vi "Create Startup CDF (Software Set).vi"(3 "Application Path":path, 4 "Add-ons":T1[](array[typedef]) {"component type" items=["standard", "hidden", "system", "unknown", "startup", "image", "essential"]}, 5 "Device Class":string, 6 "Software Set":T1 {"component type" items=["standard", "hidden", "system", "unknown", "startup", "image", "essential"]}, 7 "Operating System":string, 8 "error in (no error)":errorcluster, 9 "Files":path[](array[path]), 10 "Application Info":T1={"title"="", "description"="", "ID"="", "version"="", "component type"=4} {"component type" items=["standard", "hidden", "system", "unknown", "startup", "image", "essential"]}, 11 "CDF Location":path) -> (0 "error out":errorcluster)   [LabVIEW 2017, in "nisyscfg.lvlib"]
uses:
  <vilib>/nisyscfg/nisyscfg.lvlib
  <vilib>/nisyscfg/Software 1.2.ctl
  <vilib>/nisyscfg/Component Type.ctl
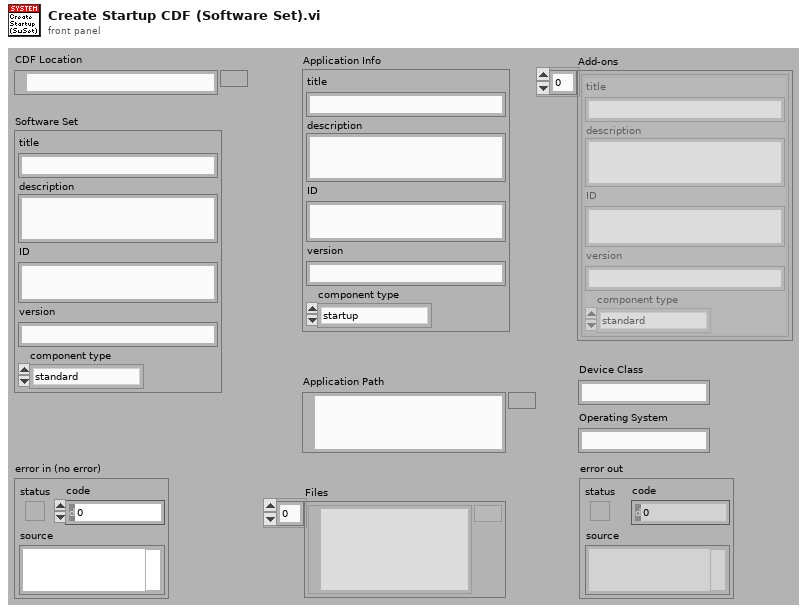
[diagram p1: front panel]
types:
  T1 = typedef "nisyscfg.lvlib/Software 1.2.ctl" = cluster{"title":string, "description":string, "ID":string, "version":string, "component type":T2}
  T2 = typedef "nisyscfg.lvlib/Component Type.ctl" = u32
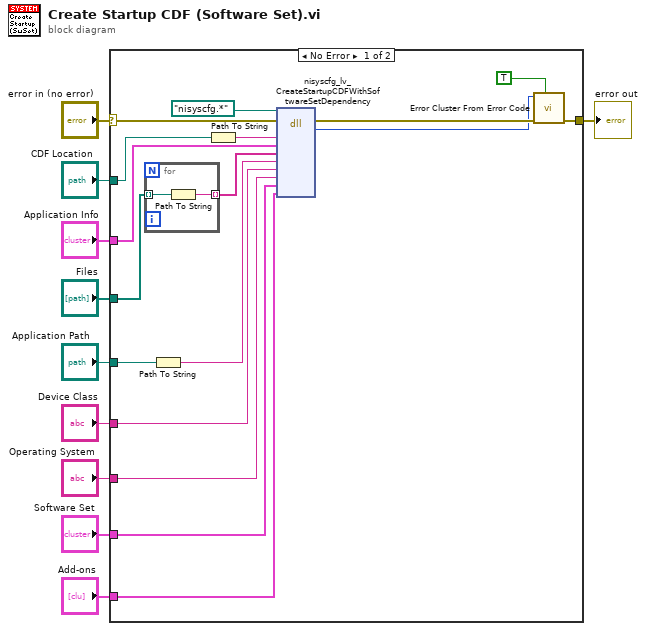
[diagram p0: block diagram]
diagram:
  n1 = case shown="No Error" "error in (no error)" {
    selector: "error in (no error)" -> [w23 w30]
    tunnel: [w22 w30] -> w9
    tunnel: "CDF Location" -> [w21 _]
    tunnel: "Application Info" -> [w16 _]
    tunnel: "Files" -> [w15 _]
    tunnel: "Device Class" -> [w19 _]
    tunnel: "Operating System" -> [w18 _]
    tunnel: "Add-ons" -> [w17 _]
    tunnel: "Software Set" -> [w13 _]
    tunnel: "Application Path" -> [w12 _]
    frame No Error {
      n2 = for {
        tunnel: w15 -> [w29] mode=indexing
        tunnel: [w28] -> w14 mode=indexing
        n3 = Path To String(path=w29) -> (string=w28:string)
      }
      n4 = Path To String(path=w12) -> (string=w11:string)
      n5 = Path To String(path=w21) -> (string=w20:string)
      n6 = dll-call lib="C:/projects/MAX/components/apis/trunk/5.0/objects/scs_nisyscfg_library_dynamic/win32U/i386/msvc90/debug/nisyscfg.dll" fn="nisyscfg_lv_CreateStartupCDFWithSoftwareSetDependency" label="CreateStartupCDFWithSoftwareSetDependency"(path in=path "nisyscfg.*", error in=w23, "cdfLocation"=w20, "applicationInfo"=w16, "files"=w14, "applicationPath"=w11, "deviceClass"=w19, "operatingSystem"=w18, "softwareSetInfo"=w13, "addons"=w17) -> (error out=w27:errorcluster, "result"=w26:i32)  [unwired: 9 in, 1 out]
      n7 = call <vilib>:"Error Cluster From Error Code.vi"("show call chain? (False)"=TRUE, "error in (no error)"=w27, "error code (0)"=w26) -> ("error out"=w22:errorcluster)  [unwired: 6 in]
    }
    frame Error {
    }
  }
  "error out" <- w9
